vi "Open Excel Template.vi"(8 "error in (no error)":errorcluster, 11 "Patrimonio":string) -> (0 "error out":errorcluster, 3 "new path":path)   [LabVIEW 2015]
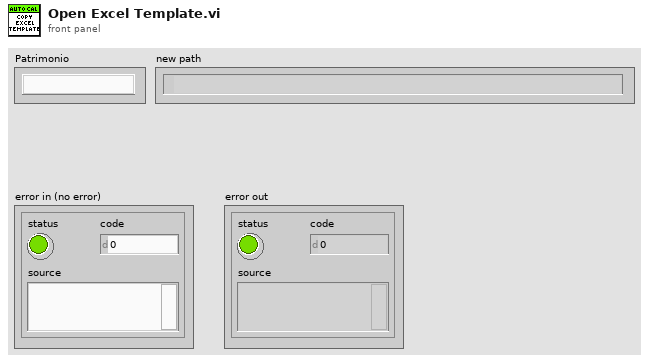
[diagram p1: front panel]
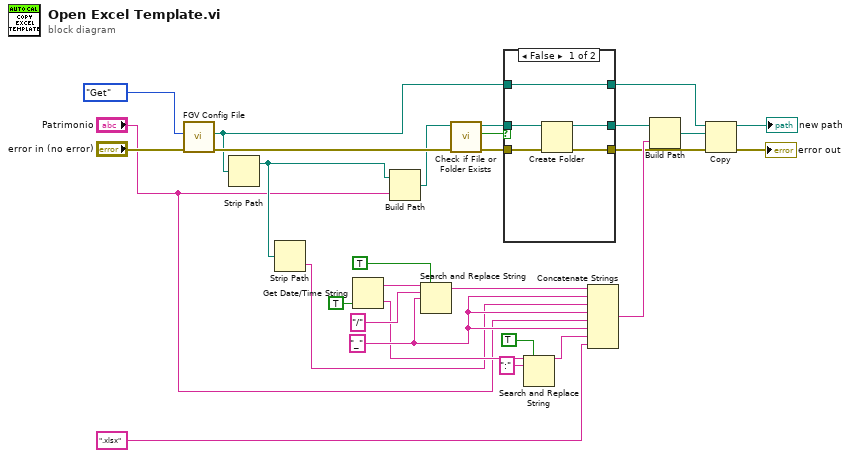
[diagram p0: block diagram]
diagram:
  w9 = "_" ("replace string (\"\")")
  n1 = call "FGV Config File.vi"("Error In"="error in (no error)", "Set/Get"=enum16{"Get", "Set"}."Get") -> ("Error Out"=w18:errorcluster, "Template File"=w11:path)  [unwired: 7 in, 1 out]
  n2 = Strip Path(path=w11) -> (stripped path=w3:path)  [unwired: 1 out]
  n3 = Strip Path(path=w3) -> (name=w2:string)  [unwired: 1 out]
  n4 = Get Date/Time String(want seconds? (F)=TRUE) -> (date string=w24:string, time string=w7:string)  [unwired: 2 in]
  n5 = Build Path(base path=w3, name or relative path="Patrimonio") -> (appended path=w12:path)
  n6 = Search and Replace String(replace all?=TRUE ("replace all? (F)"), input string=w24, search string="/", replace string=w9) -> (result string=w21:string)  [unwired: 4 in, 3 out]
  n7 = call <vilib>:"Check if File or Folder Exists.vi"("error in (no error)"=w18, "path"=w12) -> ("error out"=w15:errorcluster, "file or folder exists?"=w13:bool, "dup path"=w14:path)  [unwired: 7 in]
  n8 = case shown="False" w13 {
    tunnel: w14 -> [w33 w35]
    tunnel: w15 -> [w34 w36]
    tunnel: [w32 w36] -> w16
    tunnel: [w31 w37] -> w20
    tunnel: w11 -> [w31 w37]
    tunnel: [w30 w35] -> w25
    frame False {
      n9 = Create Folder(path (use dialog)=w33, error in=w34) -> (created path=w30:path, error out=w32:errorcluster)  [unwired: 1 in, 1 out]
    }
    frame True {
    }
  }
  n10 = Search and Replace String(replace all?=TRUE ("replace all? (F)"), input string=w7, search string=":") -> (result string=w5:string)  [unwired: 5 in, 3 out]
  n11 = Concatenate Strings(w21, w9, w2, w9, "Patrimonio", w9, w5, ".xlsx" ("string")) -> (w26:string)
  n12 = Build Path(base path=w25, name or relative path=w26) -> (appended path=w27:path)
  n13 = Copy(8:w16, 10:w27, 11:w20) -> (0:→"error out":errorcluster, 3:→"new path":path)  [unwired: 2 in, 1 out]
